vi "Process File.vi"(8 "error in (no error)":errorcluster, 10 "Result in":refnum<class "Acquired Result.lvclass">, 11 "Format Resonances in":refnum<class "Format Resonances.lvclass">) -> (0 "error out":errorcluster, 2 "Result out":refnum<class "Acquired Result.lvclass">, 3 "Format Resonances out":refnum<class "Format Resonances.lvclass">)   [LabVIEW 2018, in "Format Resonances.lvclass"]
uses:
  Format Resonances.lvclass
  NHMFL_Core/Libraries/Instruments/Results/Acquired Result/Acquired Result.lvclass
  Format Resonances.lvclass/Format Resonances.ctl
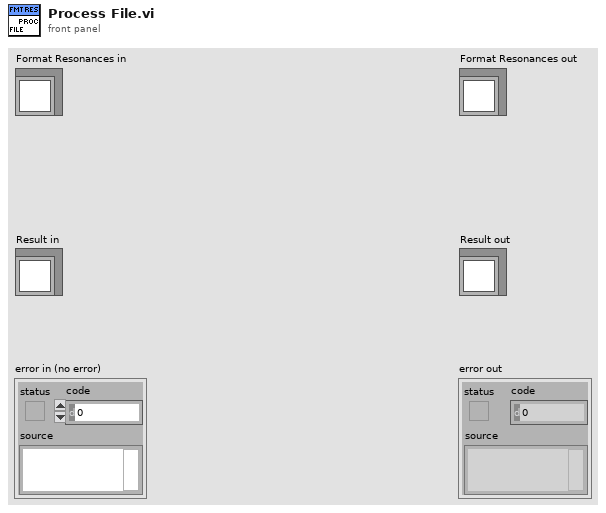
[diagram p1: front panel]
types:
  T1 = enum16{"open", "open or create", "create or replace", "create", "open (read-only)"}
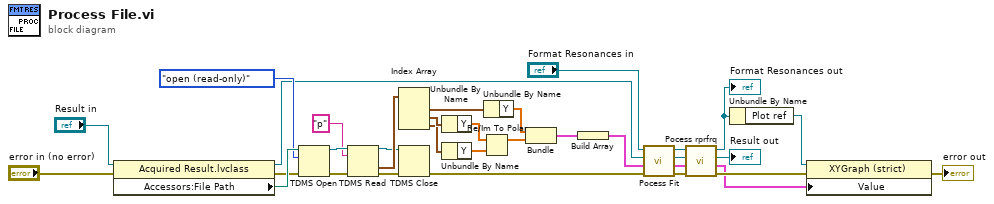
[diagram p0: block diagram]
diagram:
  n1 = property class="Acquired Result.lvclass"(reference="Result in", error in="error in (no error)") -> (reference out=w23:refnum<class "Acquired Result.lvclass">, error out=w21:errorcluster, "Accessors:File Path"=w31:path)
  n2 = TDMS Open(8:w21, 10:T1."open (read-only)" ("operation (0:open)"), 11:w31) -> (0:w28:errorcluster, 3:w29:refnum<k34>)  [unwired: 4 in]
  n3 = TDMS Read(0:w29, 5:"p" ("group name in"), 11:w28) -> (4:w25:refnum<k34>, 10:w26:waveform(dbl)[], 15:w24:errorcluster)  [unwired: 5 in, 3 out]
  n4 = Index Array(array=w26) -> (element #1=w20:waveform(dbl), element #2=w19:waveform(dbl), element #3=w18:waveform(dbl))  [unwired: 3 in]
  n5 = TDMS Close(8:w24, 11:w25) -> (0:w8:errorcluster)  [unwired: 1 out]
  n6 = Unbundle By Name(w19) -> ("Y"=w17:dbl[])
  n7 = Unbundle By Name(w18) -> ("Y"=w16:dbl[])
  n8 = Re/Im To Polar(2:w16, 3:w17) -> (1:w14:dbl[])  [unwired: 1 out]
  n9 = Unbundle By Name(w20) -> ("Y"=w15:dbl[])
  n10 = Bundle("Y"=w15, w14) -> (w12:cluster{"Y":dbl[], dbl[]})  [unwired: 1 in]
  n11 = Build Array(w12) -> (w10:cluster{"Y":dbl[], dbl[]}[])
  n12 = call-dynamic "Pocess Fit.vi"("error in (no error)"=w8, "Plot in"=w10, "Result in"=w23, "Format Resonances in"="Format Resonances in") -> ("error out"=w9:errorcluster, "Plot out"=w2:cluster{dbl[], dbl[]}[], "Result out"=w4:refnum<class "Acquired Result.lvclass">, "Format Resonances out"=w6:refnum<class "Format Resonances.lvclass">)  [unwired: 4 in]
  n13 = call-dynamic "Pocess rprfrq.vi"("error in (no error)"=w9, "Plot in"=w2, "Result in"=w4, "Format Resonances in"=w6) -> ("error out"=w7:errorcluster, "Plot out"=w1:cluster{dbl[], dbl[]}[], "Result out"=→"Result out":refnum<class "Acquired Result.lvclass">, "Format Resonances out"=w5:refnum<class "Format Resonances.lvclass">)  [unwired: 4 in]
  "Format Resonances out" <- w5
  n14 = Unbundle By Name(w5) -> ("Plot ref"=w13:refnum<vi>)
  n15 = property class="XYGraph (strict)"(reference=w13, error in=w7, "Value"=w1) -> (error out=→"error out":errorcluster)  [unwired: 1 out]
